vi "logger_make_log_data.vi"(2 "Data":string, 3 "Msg":string, 4 "Sender":string) -> (0 "log data":string)   [LabVIEW 2019]
doc: "Combines sender, msg, and data to tab-separated spreadsheet-friendly string:\n<optional timestamp> <sender> <msg> <data>\n\nEach line ended with a line feed (\"\\n\")"
panel:
  in  "add ts?":bool=TRUE
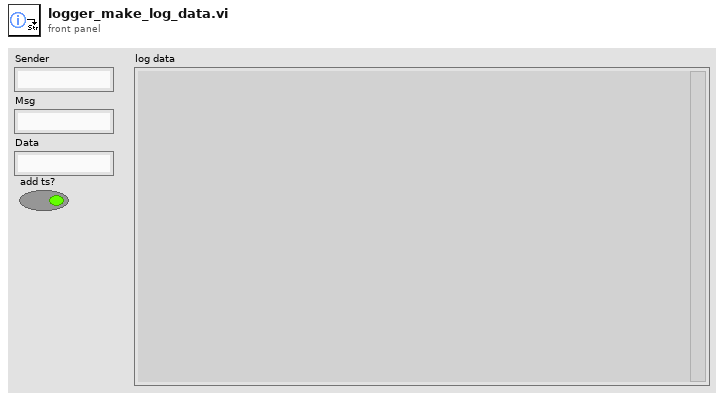
[diagram p1: front panel]
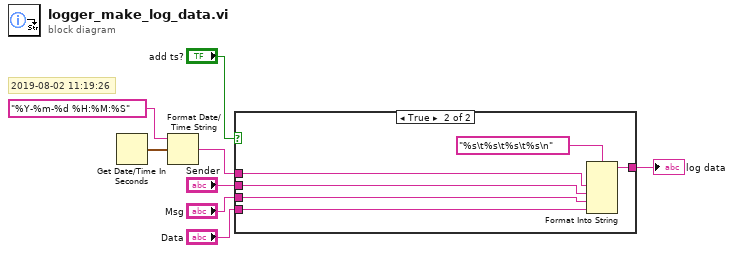
[diagram p0: block diagram]
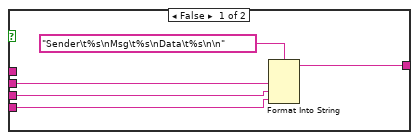
[diagram p2: hidden frame]
diagram:
  # "2019-08-02 11:19:26"
  n1 = Get Date/Time In Seconds() -> (seconds since 1Jan1904=w8:timestamp)
  n2 = Format Date/Time String(time format string (%c)="%Y-%m-%d %H:%M:%S", seconds (now)=w8) -> (date/time string=w6:string)  [unwired: 1 in]
  n3 = case shown="True" "add ts?" {
    tunnel: w6 -> [_ w18]
    tunnel: "Sender" -> [w11 w17]
    tunnel: "Msg" -> [w10 w16]
    tunnel: "Data" -> [w9 w15]
    tunnel: [w12 w14] -> w2
    frame False {
      n4 = Format Into String(format string="Sender\t%s\nMsg\t%s\nData\t%s\n\n", w11, w10, w9) -> (resulting string=w12:string)  [unwired: 2 in, 1 out]
    }
    frame True {
      n5 = Format Into String(format string="%s\t%s\t%s\t%s\n", w18, w17, w16, w15) -> (resulting string=w14:string)  [unwired: 2 in, 1 out]
    }
  }
  "log data" <- w2
